vi "c ctre phoenix get status string.vi"(8 "error in (no error)":errorcluster, 11 "statusCode":i32) -> (0 "error out":errorcluster, 2 "toFill out":string)   [LabVIEW 2020, in "CTRE_PhoenixTools.lvlib"]
doc: "CTREXPORT void c_ctre_phoenix_get_status_string(int statusCode, char *toFill, uint32_t toFillLength);"
uses:
  CTRE_PhoenixTools.lvlib
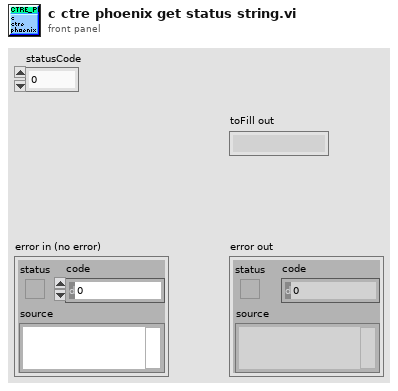
[diagram p1: front panel]
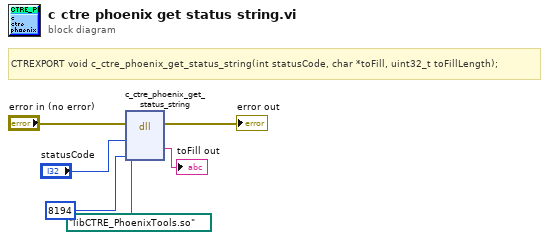
[diagram p0: block diagram]
diagram:
  # "CTREXPORT void c_ctre_phoenix_get_status_string(int statusCode, char *toFill, uint32_t toFillLength);"
  n1 = dll-call lib="?" fn="c_ctre_phoenix_get_status_string"(path in=path "libCTRE_PhoenixTools.so", error in="error in (no error)", "statusCode"="statusCode", "toFillLength"=u32 8194) -> (error out=→"error out":errorcluster, "toFill"=→"toFill out":string)  [unwired: 5 in, 1 out]
